vi "Write Command and Read.vi"(5 "Wait before read (0ms)":u32, 6 "error in (no error)":errorcluster, 7 "Bytes to read (100)":u32=100, 8 "Command":string, 9 "VISA resource name":refnum<visa-resource-name>="COM5") -> (0 "error out":errorcluster={"status"=TRUE, "code"=-1073807339, "source"="VISA Read dans Newport ESP301.lvlib:Write Command and Read.vi"}, 2 "Returned string":string, 3 "VISA resource name out":refnum<visa-resource-name>="COM5")   [LabVIEW 2011]
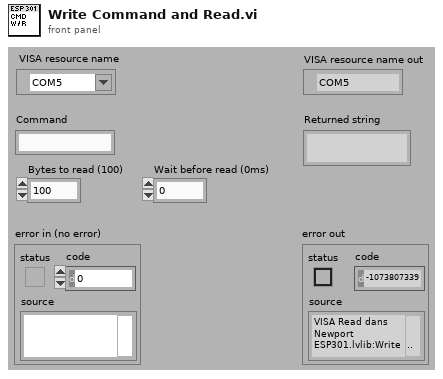
[diagram p1: front panel]
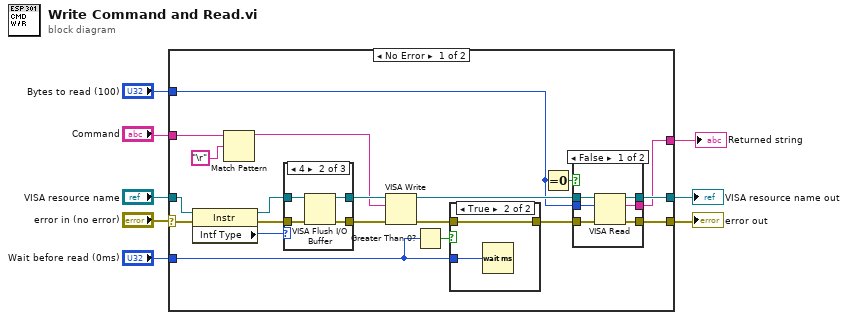
[diagram p0: block diagram]
diagram:
  n1 = case shown="No Error" "error in (no error)" {
    selector: "error in (no error)" -> [w13 w49]
    tunnel: [w28 w49] -> w7
    tunnel: "VISA resource name" -> [w15 w48]
    tunnel: [w26 w48] -> w5
    tunnel: "Command" -> [w11 _]
    tunnel: "Bytes to read (100)" -> [w18 _]
    tunnel: [w25 _] -> w2
    tunnel: "Wait before read (0ms)" -> [w20 _]
    frame No Error {
      n2 = property class="Instr"(reference=w15, error in=w13) -> (reference out=w14:refnum<visa-resource-name>, error out=w12:errorcluster, "Intf Type"=w16:u16)
      n3 = Match Pattern(string=w11, regular expression="\r") -> (before substring=w9:string)  [unwired: 4 out]
      n4 = case shown="4" w16 {
        tunnel: w14 -> [w30 w32 w36]
        tunnel: [w30 w31 w36] -> w24
        tunnel: w12 -> [w29 w34 w35]
        tunnel: [w29 w33 w35] -> w23
        frame 1 {
        }
        frame 4 {
          n5 = VISA Flush I/O Buffer(VISA resource name=w32, error in (no error)=w34) -> (VISA resource name out=w31:refnum<visa-resource-name>, error out=w33:errorcluster)  [unwired: 1 out]
        }
        frame Default {
        }
      }
      n6 = VISA Write(VISA resource name=w24, write buffer=w9, error in (no error)=w23) -> (VISA resource name out=w27:refnum<visa-resource-name>, error out=w22:errorcluster)  [unwired: 1 out]
      n7 = Greater Than 0?(x=w20) -> (x > 0?=w19:bool)
      n8 = case shown="True" w19 {
        tunnel: w22 -> [w45 w47]
        tunnel: [w45 w47] -> w21
        tunnel: w20 -> [_ w46]
        frame False {
        }
        frame True {
          n9 = Wait (ms)(milliseconds to wait=w46) -> ()  [unwired: 1 out]
        }
      }
      n10 = Equal To 0?(x=w18) -> (x = 0?=w17:bool)
      n11 = case shown="False" w17 {
        tunnel: [w42 w44] -> w28
        tunnel: w27 -> [w41 w43]
        tunnel: [w40 w43] -> w26
        tunnel: w18 -> [w39 _]
        tunnel: [w38 _] -> w25
        tunnel: w21 -> [w37 w44]
        frame False {
          n12 = VISA Read(VISA resource name=w41, byte count=w39, error in (no error)=w37) -> (VISA resource name out=w40:refnum<visa-resource-name>, read buffer=w38:string, error out=w42:errorcluster)  [unwired: 1 out]
        }
        frame True {
        }
      }
    }
    frame Error {
    }
  }
  "error out" <- w7
  "VISA resource name out" <- w5
  "Returned string" <- w2
